vi "步态方向转换 (子VI).vi"(10 "速度":i32, 11 "Gait":i8(ring)=-1 items=["Stop"=-1, "Right translation"=6, "Back translation"=12, "Turning right"=0, "Turning left"=15, "Forward translation"=3, "Left translation"=9, "Gyro rotating"=16]) -> (3 "输出":dbl[](array[numeric]))   [LabVIEW 2017]
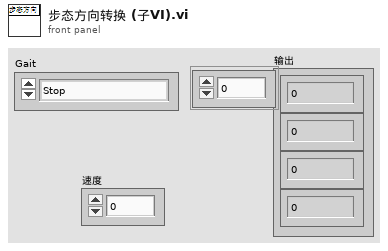
[diagram p1: front panel]
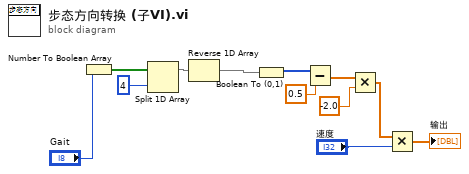
[diagram p0: block diagram]
diagram:
  n1 = Number To Boolean Array(number="Gait") -> (Boolean array=w5:bool[])
  n2 = Split 1D Array ("拆分一维数组")(array=w5, index=4 ("索引")) -> (first subarray=w6:bool[])  [unwired: 1 out]
  n3 = Reverse 1D Array(array=w6) -> (reversed array=w7:bool[])
  n4 = Boolean To (0,1)(Boolean=w7) -> (0, 1=w8:i16[])
  n5 = Subtract(x=w8, y=0.5) -> (x-y=w10:dbl[])
  n6 = Multiply(x=w10, y=-2.0) -> (x*y=w12:dbl[])
  n7 = Multiply(x=w12, y="速度") -> (x*y=→"输出":dbl[])
